vi "Actor Core.vi"(8 "error in":errorcluster, 11 "PowerSupply in":refnum<class "PowerSupply.lvclass">) -> (0 "error out":errorcluster, 3 "Actor out":refnum<class "Actor.lvclass">)   [LabVIEW 2019, in "PowerSupply.lvlib" / "PowerSupply.lvclass"]
doc: "The instrument actor core is only here to distribute panel resolution settings to children classes."
uses:
  Library/PowerSupply.lvclass
  C:/Users/Public/Documents/Development/builds/Instruments/Instruments.lvlibp/Library/Instruments.lvclass
  builds/Engine/Actor Framework.lvlibp/1abvi3w/vi.lib/ActorFramework/Actor/Actor.lvclass
  Custom Controls/Settings.ctl
  Custom Controls/Sense Point.ctl
  Custom Controls/OCP Mode.ctl
  Custom Controls/Status_Flags.ctl
  Library/PowerSupply.lvclass/PowerSupply.ctl
  PowerSupply Messages/Write Voltage Msg/Write Voltage Msg.lvclass/Write Voltage Msg.ctl
  PowerSupply Messages/Write Current Msg/Write Current Msg.lvclass/Write Current Msg.ctl
  PowerSupply Messages/Write Limit Current Msg/Write Limit Current Msg.lvclass/Write Limit Current Msg.ctl
  PowerSupply Messages/Write Limit Volt Msg/Write Limit Volt Msg.lvclass/Write Limit Volt Msg.ctl
  PowerSupply Messages/Write Ramp Volt Msg/Write Ramp Volt Msg.lvclass/Write Ramp Volt Msg.ctl
  PowerSupply Messages/Write Ramp Current Msg/Write Ramp Current Msg.lvclass/Write Ramp Current Msg.ctl
  PowerSupply Messages/Write Output_Enable Msg/Write Output_Enable Msg.lvclass/Write Output_Enable Msg.ctl
  PowerSupply Messages/Write OVP_Enable Msg/Write OVP_Enable Msg.lvclass/Write OVP_Enable Msg.ctl
  PowerSupply Messages/Write OCP_Enable Msg/Write OCP_Enable Msg.lvclass/Write OCP_Enable Msg.ctl
  PowerSupply Messages/Write Interlock_Enable Msg/Write Interlock_Enable Msg.lvclass/Write Interlock_Enable Msg.ctl
  PowerSupply Messages/Write Current_Share Msg/Write Current_Share Msg.lvclass/Write Current_Share Msg.ctl
  PowerSupply Messages/Write Sense_Point Msg/Write Sense_Point Msg.lvclass/Write Sense_Point Msg.ctl
  PowerSupply Messages/Write OCP_Mode Msg/Write OCP_Mode Msg.lvclass/Write OCP_Mode Msg.ctl
  PowerSupply Messages/Write Active Channel Msg/Write Active Channel Msg.lvclass/Write Active Channel Msg.ctl
  Accessors/Write Measured Table.vi
  Accessors/Write Channel Ring.vi
  Accessors/Write Settings_Ref.vi
  Accessors/Write Status_Ref.vi
  builds/Instruments/Instruments.lvlibp/Accessors/Write Graph_Ref.vi
  builds/Engine/Actor Framework.lvlibp/1abvi3w/vi.lib/ActorFramework/Message Enqueuer/Enqueue.vi
  PowerSupply Messages/Reset Supply Msg/Reset Supply Msg.lvclass
  PowerSupply Messages/Synch From Supply Msg/Synch From Supply Msg.lvclass
  PowerSupply Messages/Write Voltage Msg/Write Voltage Msg.lvclass
  PowerSupply Messages/Write Current Msg/Write Current Msg.lvclass
  PowerSupply Messages/Write Limit Current Msg/Write Limit Current Msg.lvclass
  PowerSupply Messages/Write Limit Volt Msg/Write Limit Volt Msg.lvclass
  PowerSupply Messages/Write Ramp Volt Msg/Write Ramp Volt Msg.lvclass
  PowerSupply Messages/Write Ramp Current Msg/Write Ramp Current Msg.lvclass
  PowerSupply Messages/Write Output_Enable Msg/Write Output_Enable Msg.lvclass
  PowerSupply Messages/Write OVP_Enable Msg/Write OVP_Enable Msg.lvclass
  PowerSupply Messages/Write OCP_Enable Msg/Write OCP_Enable Msg.lvclass
  PowerSupply Messages/Write Interlock_Enable Msg/Write Interlock_Enable Msg.lvclass
  PowerSupply Messages/Write Current_Share Msg/Write Current_Share Msg.lvclass
  PowerSupply Messages/Write Sense_Point Msg/Write Sense_Point Msg.lvclass
  PowerSupply Messages/Write OCP_Mode Msg/Write OCP_Mode Msg.lvclass
  PowerSupply Messages/Write Active Channel Msg/Write Active Channel Msg.lvclass
  builds/Instruments/Instruments.lvlibp/Library/Instruments.lvclass
panel:
  out "Status":T1
  in  "Active Device":u16(ring)
  in  "Sync":bool
  in  "Reset":bool
  in  "View":enum16{"Graph", "Table"}(ring)
  in  "Channel":u16(ring)
  out "Display Format":enum32{"Graph", "Table"}(tab)
  out "Waveform Chart":waveform(dbl)[](graph)
  out "Measured Table":i32(listbox)
  in  "Settings":T2
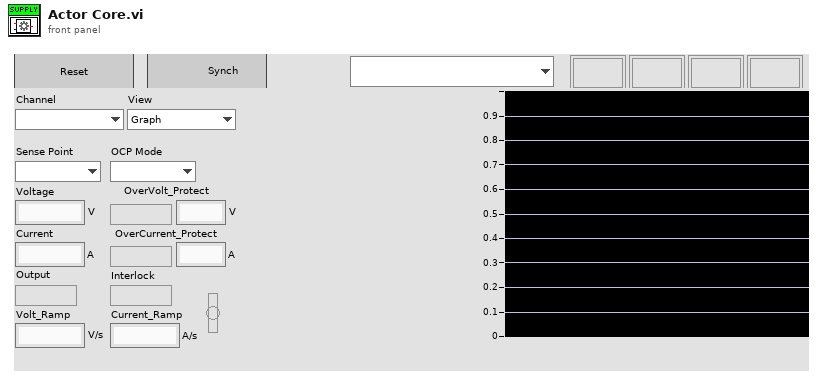
[diagram p1: front panel]
types:
  T1 = typedef "PowerSupply.lvlib/PowerSupply.lvclass/Status_Flags.ctl" = cluster{"Interlock":bool, "OVP":bool, "OCP":bool, "Output":bool}
  T2 = typedef "PowerSupply.lvlib/PowerSupply.lvclass/Settings.ctl" = cluster{"Voltage":dbl, "Current":dbl, "Output":bool, "OverVolt_Protect":dbl, "OverCurrent_Protect":dbl, "OVP":bool, "OCP":bool, "Interlock":bool, "Volt_Ramp":dbl, "Current_Ramp":dbl, "Sense Point":T3, "OCP Mode":T4, "Sharing":bool}
  T3 = typedef "PowerSupply.lvlib/PowerSupply.lvclass/Sense Point.ctl" = enum16{"Local", "Remote"}
  T4 = typedef "PowerSupply.lvlib/PowerSupply.lvclass/OCP Mode.ctl" = enum16{"Shutdown", "Foldback"}
  T5 = cluster{"Pnl Actor":refnum<event-registration>, "Event Registration Refnum":refnum<event-registration>}
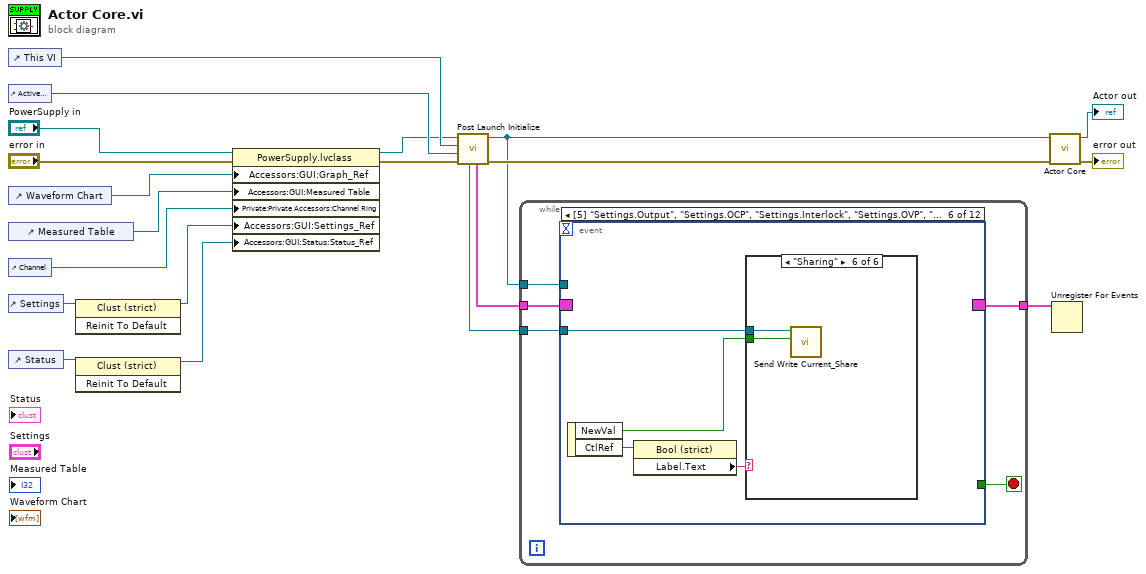
[diagram p0: block diagram]
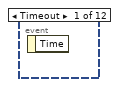
[diagram p2: hidden frame]
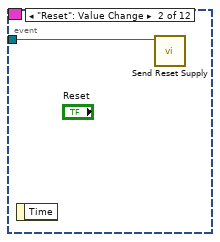
[diagram p3: hidden frame]
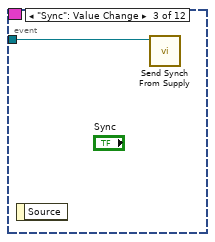
[diagram p4: hidden frame]
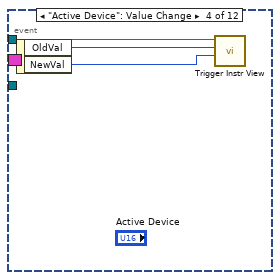
[diagram p5: hidden frame]
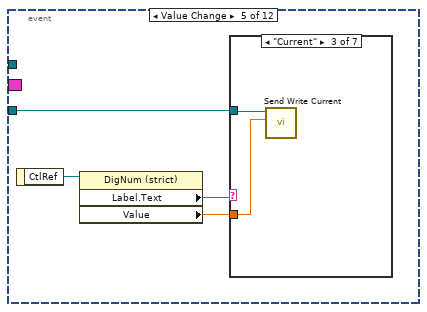
[diagram p6: hidden frame]
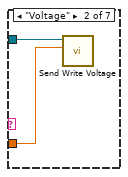
[diagram p8: hidden frame]
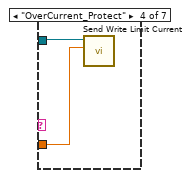
[diagram p9: hidden frame]
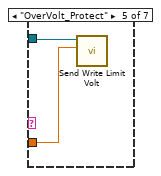
[diagram p10: hidden frame]
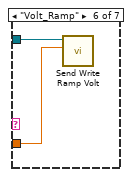
[diagram p11: hidden frame]
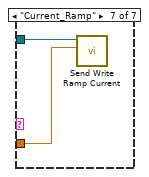
[diagram p12: hidden frame]
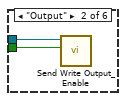
[diagram p14: hidden frame]
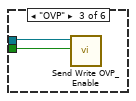
[diagram p15: hidden frame]
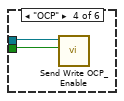
[diagram p16: hidden frame]
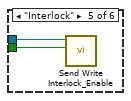
[diagram p17: hidden frame]
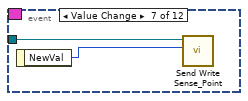
[diagram p18: hidden frame]
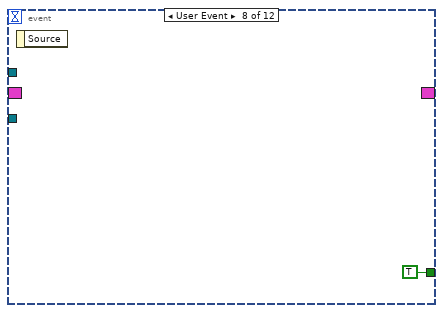
[diagram p19: hidden frame]
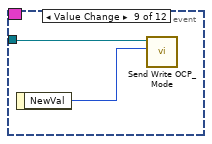
[diagram p20: hidden frame]
diagram:
  n1 = control-ref of="This VI"() -> (w16:refnum<vi>)
  n2 = control-ref of="Active Device"() -> (w14:refnum<vi>)
  n3 = control-ref of="Waveform Chart"() -> (w9:refnum<vi>)
  n4 = control-ref of="Measured Table"() -> (w8:refnum<vi>)
  n5 = control-ref of="Channel"() -> (w4:refnum<vi>)
  n6 = control-ref of="Settings"() -> (w7:refnum<vi>)
  n7 = control-ref of="Status"() -> (w2:refnum<vi>)
  n8 = invoke class="Clust (strict)" method="Reinit To Default"(reference=w7) -> (reference out=w3:refnum<vi>)  [unwired: 2 in, 2 out]
  n9 = invoke class="Clust (strict)" method="Reinit To Default"(reference=w2) -> (reference out=w1:refnum<vi>)  [unwired: 2 in, 2 out]
  n10 = property class="PowerSupply.lvclass"(reference="PowerSupply in", error in="error in", "Accessors:GUI:Graph_Ref"=w9, "Accessors:GUI:Measured Table"=w8, "Private:Private Accessors:Channel Ring"=w4, "Accessors:GUI:Settings_Ref"=w3, "Accessors:GUI:Status:Status_Ref"=w1) -> (reference out=w10:refnum<class "PowerSupply.lvclass">, error out=w11:errorcluster)
  n11 = call "Post Launch Initialize.vi"("error in"=w11, "Active Device"=w14, "GUI Reference"=w16, "Instruments in"=w10) -> ("error out"=w18:errorcluster, "Instruments out"=w5:refnum<class "PowerSupply.lvclass">, "Registered Events"=w17:T5, "Self Enqueuer"=w6:refnum<class "Message Enqueuer.lvclass">)  [unwired: 4 in]
  n12 = while {
    tunnel: w17 -> [w25]
    tunnel: [w23] -> w15
    tunnel: w6 -> [w22]
    tunnel: w5 -> [w21]
    stop <- w24 stop-if-true
    n13 = event shown="[5] \"Settings.Output\", \"Settings.OCP\", \"Settings.Interlock\", \"Settings.OVP\", \"Settings.Sharing\": Value Change" {
      selector: w25 -> [_ _ _ _ _ _ _ _ _ _ _ _]
      dyn-events: [_ _ _ _ _ _ _ _ _ _ _ _] -> w23
      timeout: _ -> [_ _ _ _ _ _ _ _ _ _ _ _]
      tunnel: [_ _ _ _ _ _ _ TRUE ("Discard?") _ _ _ w69] -> w24
      tunnel: w22 -> [_ w26 w27 _ w31 w49 w62 _ w65 w67 _ _]
      tunnel: w21 -> [_ _ _ w28 _ _ _ _ _ _ _ _]
      event Timeout {
        n14 = event-data() -> ()  [unwired: 1 in, 1 out]
      }
      event "Reset": Value Change {
        n15 = event-data() -> ()  [unwired: 1 in, 1 out]
        n16 = call "Send Reset Supply.vi"("Message Enqueuer"=w26) -> ()  [unwired: 9 in, 2 out]
      }
      event "Sync": Value Change {
        n17 = event-data() -> ()  [unwired: 1 in, 1 out]
        n18 = call "Send Synch From Supply.vi"("Message Enqueuer"=w27) -> ()  [unwired: 9 in, 2 out]
      }
      event "Active Device": Value Change {
        n19 = event-data() -> ("OldVal"=w30:u16, "NewVal"=w29:u16)  [unwired: 1 in]
        n20 = call "Trigger Instr View.vi"("New Value"=w29, "Old Value"=w30, "Instruments in"=w28) -> ()  [unwired: 7 in, 2 out]
      }
      event Value Change {
        n21 = event-data() -> ("CtlRef"=w34:refnum<vi>)  [unwired: 1 in]
        n22 = property class="DigNum (strict)"(reference=w34) -> ("Label.Text"=w33:string, "Value"=w32:dbl)  [unwired: 1 in, 2 out]
        n23 = case shown="\"Current\"" w33 {
          tunnel: w32 -> [_ w35 w37 w39 w41 w43 w45]
          tunnel: w31 -> [_ w36 w38 w40 w42 w44 w46]
          frame "False", Default {
          }
          frame "Voltage" {
            n24 = call "Send Write Voltage.vi"("Voltage"=w35, "Message Enqueuer"=w36) -> ()  [unwired: 8 in, 2 out]
          }
          frame "Current" {
            n25 = call "Send Write Current.vi"("Current"=w37, "Message Enqueuer"=w38) -> ()  [unwired: 8 in, 2 out]
          }
          frame "OverCurrent_Protect" {
            n26 = call "Send Write Limit Current.vi"("OverCurrent_Protect"=w39, "Message Enqueuer"=w40) -> ()  [unwired: 8 in, 2 out]
          }
          frame "OverVolt_Protect" {
            n27 = call "Send Write Limit Volt.vi"("OverVolt_Protect"=w41, "Message Enqueuer"=w42) -> ()  [unwired: 8 in, 2 out]
          }
          frame "Volt_Ramp" {
            n28 = call "Send Write Ramp Volt.vi"("Voltage_Ramp"=w43, "Message Enqueuer"=w44) -> ()  [unwired: 8 in, 2 out]
          }
          frame "Current_Ramp" {
            n29 = call "Send Write Ramp Current.vi"("Current_Ramp"=w45, "Message Enqueuer"=w46) -> ()  [unwired: 8 in, 2 out]
          }
        }
      }
      event Value Change {
        n30 = event-data() -> ("NewVal"=w48:bool, "CtlRef"=w50:refnum<vi>)  [unwired: 1 in]
        n31 = property class="Bool (strict)"(reference=w50) -> ("Label.Text"=w47:string)  [unwired: 1 in, 2 out]
        n32 = case shown="\"Sharing\"" w47 {
          tunnel: w49 -> [_ w52 w54 w56 w58 w60]
          tunnel: w48 -> [_ w51 w53 w55 w57 w59]
          frame "False", Default {
          }
          frame "Output" {
            n33 = call "Send Write Output_Enable.vi"("Output_Enable"=w51, "Message Enqueuer"=w52) -> ()  [unwired: 8 in, 2 out]
          }
          frame "OVP" {
            n34 = call "Send Write OVP_Enable.vi"("OVP_Enable"=w53, "Message Enqueuer"=w54) -> ()  [unwired: 8 in, 2 out]
          }
          frame "OCP" {
            n35 = call "Send Write OCP_Enable.vi"("OCP_Enable"=w55, "Message Enqueuer"=w56) -> ()  [unwired: 8 in, 2 out]
          }
          frame "Interlock" {
            n36 = call "Send Write Interlock_Enable.vi"("INTLK_Enable"=w57, "Message Enqueuer"=w58) -> ()  [unwired: 8 in, 2 out]
          }
          frame "Sharing" {
            n37 = call "Send Write Current_Share.vi"("Current_Sharing"=w59, "Message Enqueuer"=w60) -> ()  [unwired: 8 in, 2 out]
          }
        }
      }
      event Value Change {
        n38 = event-data() -> ("NewVal"=w61:T3)  [unwired: 1 in]
        n39 = call "Send Write Sense_Point.vi"("Sense Point"=w61, "Message Enqueuer"=w62) -> ()  [unwired: 8 in, 2 out]
      }
      event User Event {
        n40 = event-data() -> ()  [unwired: 1 in, 1 out]
      }
      event Value Change {
        n41 = event-data() -> ("NewVal"=w64:T4)  [unwired: 1 in]
        n42 = call "Send Write OCP_Mode.vi"("OCP Mode"=w64, "Message Enqueuer"=w65) -> ()  [unwired: 8 in, 2 out]
      }
      event "Channel": Value Change {
        n43 = event-data() -> ("NewVal"=w66:u16)  [unwired: 1 in]
        n44 = call "Send Write Active Channel.vi"("Active Channel"=w66, "Message Enqueuer"=w67) -> ()  [unwired: 8 in, 2 out]
      }
      event "View": Value Change {
        n45 = event-data() -> ()  [unwired: 1 in, 4 out]
        "Display Format" <- "View"
      }
      event Panel Close? {
        w69 = TRUE ("Discard?")
        n46 = event-data() -> ()  [unwired: 1 in, 1 out]
        n47 = event-data("Discard?"=w69) -> ()  [unwired: 1 in, 1 out]
      }
    }
  }
  n48 = call-parent "Actor Core.vi"("error in"=w18, "Instruments in"=w5) -> ("error out"=→"error out":errorcluster, "Actor out"=→"Actor out":refnum<class "Actor.lvclass">)  [unwired: 8 in]
  n49 = Unregister For Events(event registration refnum=w15) -> ()  [unwired: 1 in, 1 out]
